vi "_builtins_snap_to_panel_grid.vi"(8 "error in (no error)":errorcluster, 11 "VI Refnum in":refnum<vi>) -> (0 "error out":errorcluster, 3 "VI Refnum out":refnum<vi>)   [LabVIEW 2019, in "Script.lvlib"]
doc: "Snaps the selected front panel controls and indicators to the nearest VI panel grid size.\n\nCreated by: Ryan Pacini"
uses:
  Script.lvlib
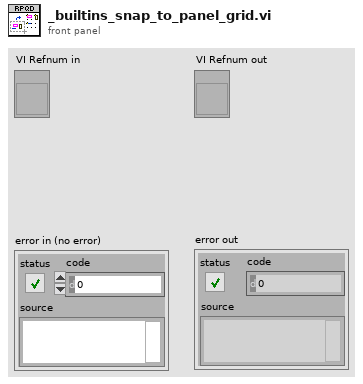
[diagram p1: front panel]
types:
  T1 = cluster{"inc_dec":bool, "label":bool, "caption":bool, "index":bool}[]
  T2 = typedef "LVRectTypeDef.ctl" = cluster{"Left":i16, "Top":i16, "Right":i16, "Bottom":i16}
  T3 = cluster{"Left":i32, "Top":i32, "Right":i32, "Bottom":i32}
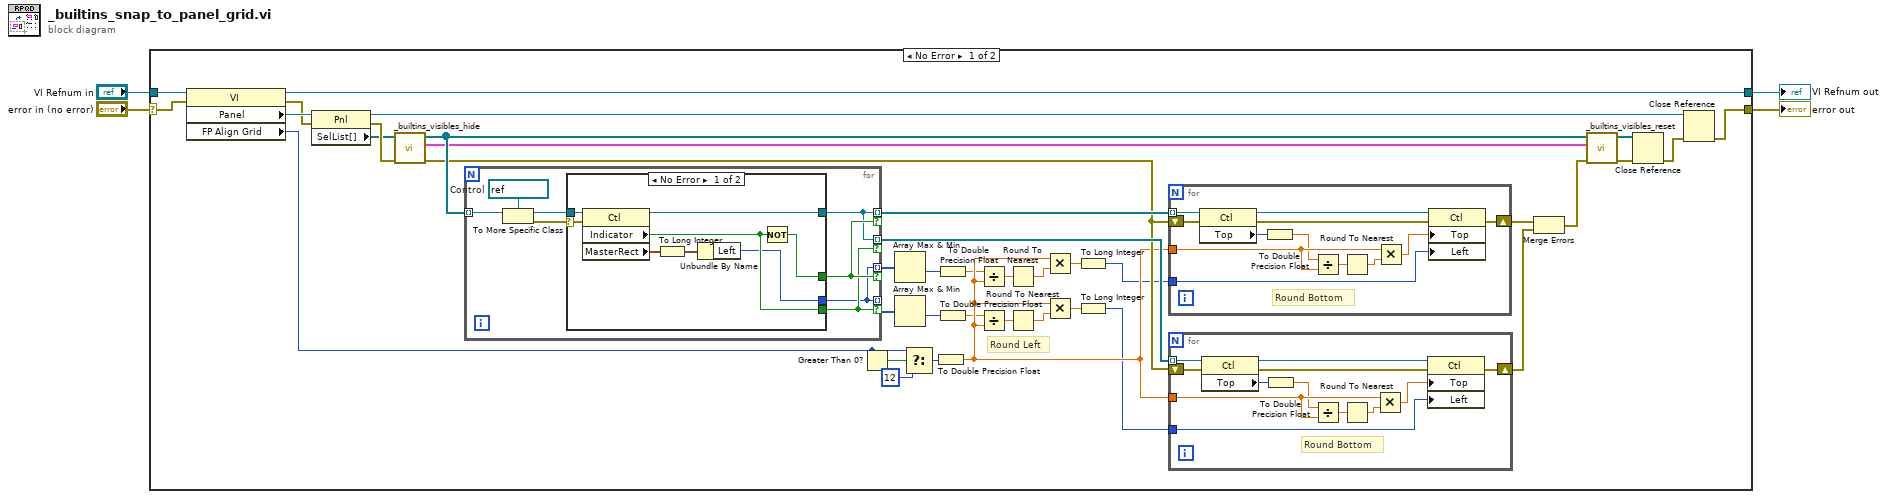
[diagram p0: block diagram]
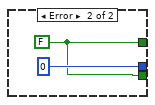
[diagram p2: hidden frame]
diagram:
  n1 = case shown="No Error" "error in (no error)" {
    selector: "error in (no error)" -> [w41 w86]
    tunnel: "VI Refnum in" -> [w39 w87]
    tunnel: [w43 w87] -> w3
    tunnel: [w42 w86] -> w2
    frame No Error {
      # "Round Left"
      n2 = property class="VI"(reference=w39, error in=w41) -> (reference out=w43:refnum<vi>, error out=w35:errorcluster, "Panel"=w40:refnum<vi>, "FP Align Grid"=w36:i32)
      n3 = property class="Pnl"(reference=w40, error in=w35) -> (reference out=w31:refnum<vi>, error out=w25:errorcluster, "SelList[]"=w24:refnum<vi>[])
      n4 = call "_builtins_visibles_hide.vi"("error in (no error)"=w25, "GObjects in"=w24) -> ("error out"=w15:errorcluster, "Reset Visible"=w21:T1, "GObjects out"=w22:refnum<vi>[])  [unwired: 7 in]
      n5 = for {
        tunnel: w22 -> [w51] mode=indexing
        tunnel: [w47] -> w32 mode=indexing if=w50
        tunnel: [w48] -> w34 mode=indexing if=w50
        tunnel: [w48] -> w33 mode=indexing if=w49
        tunnel: [w47] -> w18 mode=indexing if=w49
        w45 = refnum<vi> refnum  # Control
        n6 = To More Specific Class(target class=w45, reference=w51) -> (specific class reference=w46:refnum<vi>, error out=w44:errorcluster)  [unwired: 1 in]
        n7 = case shown="No Error" w44 {
          selector: w44 -> [w53 _]
          tunnel: [w59 w60] -> w50
          tunnel: [w58 w60] -> w49
          tunnel: [w56 0 ("Left")] -> w48
          tunnel: [w55 _] -> w47
          tunnel: w46 -> [w54 _]
          frame No Error {
            n8 = property class="Ctl"(reference=w54, error in=w53) -> (reference out=w55:refnum<vi>, "Indicator"=w58:bool, "MasterRect"=w57:T2)  [unwired: 1 out]
            n9 = To Long Integer(number=w57) -> (32bit integer=w52:T3)
            n10 = Unbundle By Name(w52) -> ("Left"=w56:i32)
            n11 = Not(x=w58) -> (.not. x?=w59:bool)
          }
          frame Error {
            w60 = FALSE
          }
        }
      }
      n12 = Greater Than 0?(x=w36) -> (x > 0?=w38:bool)
      n13 = Array Max & Min(array=w34) -> (min value=w30:i32)  [unwired: 3 out]
      n14 = Array Max & Min(array=w33) -> (min value=w29:i32)  [unwired: 3 out]
      n15 = Select(t=w36, s=w38, f=12) -> (s? t:f=w17:i32)
      n16 = To Double Precision Float(number=w17) -> (double precision float=w11:dbl)
      n17 = To Double Precision Float(number=w30) -> (double precision float=w9:dbl)
      n18 = To Double Precision Float(number=w29) -> (double precision float=w10:dbl)
      n19 = Divide(x=w9, y=w11) -> (x/y=w28:dbl)
      n20 = Divide(x=w10, y=w11) -> (x/y=w26:dbl)
      n21 = Round To Nearest(number=w28) -> (nearest integer value=w7:dbl)
      n22 = Round To Nearest(number=w26) -> (nearest integer value=w8:dbl)
      n23 = Multiply(x=w11, y=w7) -> (x*y=w27:dbl)
      n24 = Multiply(x=w11, y=w8) -> (x*y=w16:dbl)
      n25 = To Long Integer(number=w27) -> (32bit integer=w6:i32)
      n26 = To Long Integer(number=w16) -> (32bit integer=w5:i32)
      n27 = for {
        tunnel: w32 -> [w85] mode=indexing
        tunnel: w6 -> [w76]
        shift-right: [w82] -> w14
        shift-left: w15 -> [w83]
        tunnel: w11 -> [w78]
        # "Round Bottom"
        n28 = property class="Ctl"(reference=w85, error in=w83) -> (reference out=w81:refnum<vi>, error out=w84:errorcluster, "Top"=w79:i32)
        n29 = To Double Precision Float(number=w79) -> (double precision float=w75:dbl)
        n30 = Divide(x=w75, y=w78) -> (x/y=w80:dbl)
        n31 = Round To Nearest(number=w80) -> (nearest integer value=w74:dbl)
        n32 = Multiply(x=w78, y=w74) -> (x*y=w77:dbl)
        n33 = property class="Ctl"(reference=w81, error in=w84, "Top"=w77, "Left"=w76) -> (error out=w82:errorcluster)  [unwired: 1 out]
      }
      n34 = for {
        tunnel: w18 -> [w73] mode=indexing
        tunnel: w5 -> [w64]
        shift-right: [w70] -> w13
        shift-left: w15 -> [w71]
        tunnel: w11 -> [w66]
        # "Round Bottom"
        n35 = property class="Ctl"(reference=w73, error in=w71) -> (reference out=w69:refnum<vi>, error out=w72:errorcluster, "Top"=w67:i32)
        n36 = To Double Precision Float(number=w67) -> (double precision float=w63:dbl)
        n37 = Divide(x=w63, y=w66) -> (x/y=w68:dbl)
        n38 = Round To Nearest(number=w68) -> (nearest integer value=w62:dbl)
        n39 = Multiply(x=w66, y=w62) -> (x*y=w65:dbl)
        n40 = property class="Ctl"(reference=w69, error in=w72, "Top"=w65, "Left"=w64) -> (error out=w70:errorcluster)  [unwired: 1 out]
      }
      n41 = Merge Errors(w14, w13) -> (w12:errorcluster)
      n42 = call "_builtins_visibles_reset.vi"("error in (no error)"=w12, "Reset Visible"=w21, "GObjects in"=w22) -> ("error out"=w23:errorcluster, "GObjects out"=w19:refnum<vi>[])  [unwired: 7 in]
      n43 = Close Reference(reference=w19, error in (no error)=w23) -> (error out=w20:errorcluster)
      n44 = Close Reference(reference=w31, error in (no error)=w20) -> (error out=w42:errorcluster)
    }
    frame Error {
    }
  }
  "VI Refnum out" <- w3
  "error out" <- w2
